vi "4.1.1.vi"() -> ()   [LabVIEW 2018]
panel:
  in  "정지":bool
  out "웨이브폼 차트":dbl(graph)
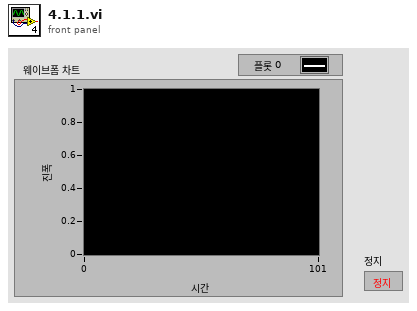
[diagram p1: front panel]
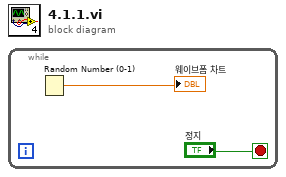
[diagram p0: block diagram]
diagram:
  n1 = while {
    stop <- "정지" stop-if-true
    n2 = Random Number (0-1)() -> (number: 0 to 1=→"웨이브폼 차트":dbl)
  }
